vi "Bernoulli Noise.vi"(7 "initialize?":bool=TRUE, 9 "seed":i32=-1, 10 "ones probability":dbl=0.5 format="%0.2f", 11 "samples":i32=128) -> (0 "error":i32, 3 "bernoulli noise":u8[](array[numeric]))   [LabVIEW 2020, in "NI_AALBase.lvlib"]
doc: "Generates a pseudorandom pattern of ones and zeros. LabVIEW computes each element of <B>bernoulli noise</B> as if flipping a coin weighted by <B>ones probability</B>."
uses:
  NI_AALBase.lvlib
panel:
  # "Bernoulli Noise"
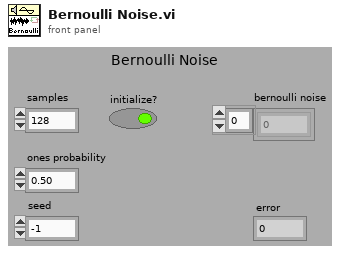
[diagram p1: front panel]
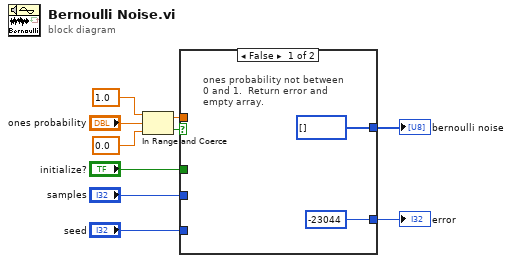
[diagram p0: block diagram]
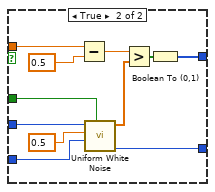
[diagram p2: hidden frame]
diagram:
  n1 = In Range and Coerce(upper limit=1.0, x="ones probability", lower limit=0.0) -> (coerced(x)=w3:dbl, In Range?=w4:bool)
  n2 = case shown="False" w4 {
    tunnel: [-23044 ("error") w23] -> w10
    tunnel: "seed" -> [_ w22]
    tunnel: "samples" -> [_ w21]
    tunnel: [i16[] [] w18] -> w7
    tunnel: w3 -> [_ w14]
    tunnel: "initialize?" -> [_ w13]
    frame False {
      # "ones probability not between \n0 and 1.  Return error and \nempty array."
    }
    frame True {
      n3 = Subtract(x=w14, y=0.5) -> (x-y=w17:dbl)
      n4 = call "Uniform White Noise.vi"("initialize?"=w13, "seed"=w22, "amplitude"=0.5, "samples"=w21) -> ("error"=w23:i32, "uniform white noise"=w15:dbl[])  [unwired: 1 in, 5 out]
      n5 = Greater?(x=w17, y=w15) -> (0:w19:bool[])
      n6 = Boolean To (0,1)(Boolean=w19) -> (0, 1=w18:i16[])
    }
  }
  "error" <- w10
  "bernoulli noise" <- w7
